vi "characteristic (SubVI).vi"(11 "Input":dbl) -> (3 "Numeric":i32)   [LabVIEW 2016]
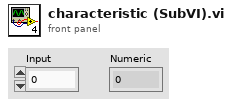
[diagram p1: front panel]
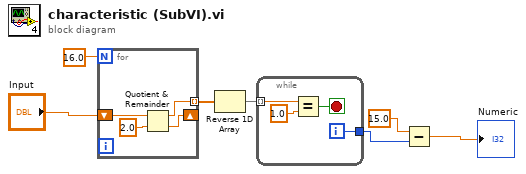
[diagram p0: block diagram]
diagram:
  n1 = for {
    N: 16.0 ("Numeric 2") -> [_]
    tunnel: [w9] -> w4 mode=indexing
    shift-right: [w8] -> _
    shift-left: "Input" -> [w11]
    n2 = Quotient & Remainder(x=w11, y=2.0) -> (x-y*floor(x/y)=w9:dbl, floor(x/y)=w8:dbl)
  }
  n3 = Reverse 1D Array(array=w4) -> (reversed array=w5:dbl[])
  n4 = while {
    tunnel: w5 -> [w15] mode=indexing
    tunnel: [w12] -> w1
    i -> [w12]
    stop <- w13 stop-if-true
    n5 = Equal?(x=w15, y=1.0) -> (x = y?=w13:bool)
  }
  n6 = Subtract(x=15.0 ("Numeric"), y=w1) -> (x-y=→"Numeric":dbl)
